vi "GetXYLocal.vi"(6 "Dummy Ref":refnum<vi>, 8 "error in (no error)":errorcluster, 10 "Global Mouse Coords":T1, 11 "Render Window in":refnum<class "Render Window.lvclass">) -> (0 "error out":errorcluster, 2 "Local Mouse Coords":T1, 3 "Render Window out":refnum<class "Render Window.lvclass">)   [LabVIEW 2015, in "Render Window.lvclass"]
uses:
  Render Window.lvclass
  3D Scene/Mouse Coords.ctl
  Render Window.lvclass/Render Window.ctl
  Input/Input.lvclass
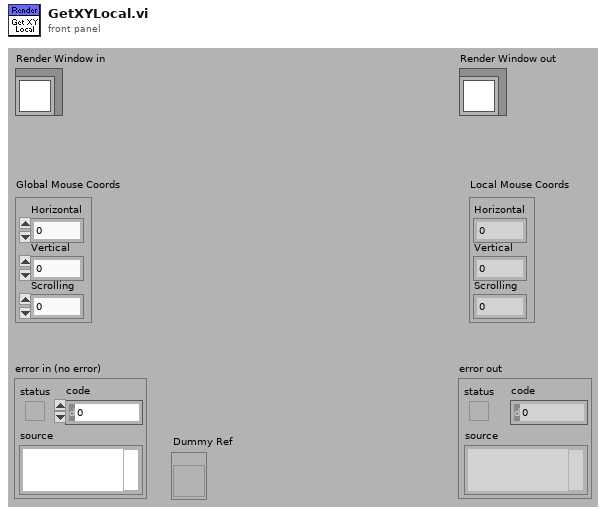
[diagram p1: front panel]
types:
  T1 = typedef "Input.lvclass/Mouse Coords.ctl" = cluster{"Horizontal":i32, "Vertical":i32, "Scrolling":i32}
  T2 = typedef "LVRectTypeDef.ctl" = cluster{"Left":i16, "Top":i16, "Right":i16, "Bottom":i16}
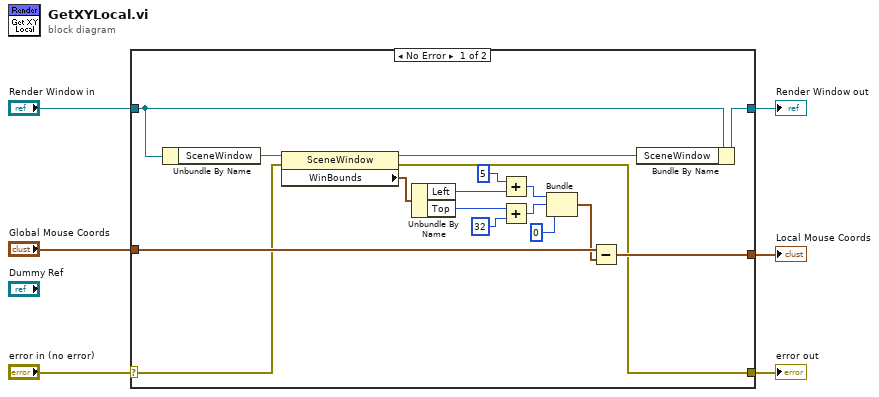
[diagram p0: block diagram]
diagram:
  n1 = case shown="No Error" "error in (no error)" {
    selector: "error in (no error)" -> [w10 w26]
    tunnel: [w9 w26] -> w5
    tunnel: [w22 w25] -> w3
    tunnel: "Render Window in" -> [w23 w25]
    tunnel: "Global Mouse Coords" -> [w13 w24]
    tunnel: [w12 w24] -> w1
    frame No Error {
      n2 = Unbundle By Name(w23) -> ("SceneWindow"=w21:refnum<vi>)
      n3 = property class="SceneWindow"(reference=w21, error in=w10) -> (reference out=w11:refnum<vi>, error out=w9:errorcluster, "WinBounds"=w20:T2)
      n4 = Unbundle By Name(w20) -> ("Left"=w19:i16, "Top"=w17:i16)
      n5 = Add(x=i16 5, y=w19) -> (x+y=w15:i16)
      n6 = Add(x=w17, y=i16 32) -> (x+y=w14:i16)
      n7 = Bundle(w15, w14, "y"=i16 0) -> (w7:cluster{i16, i16, "y":i16})  [unwired: 1 out]
      n8 = Subtract(x=w13, y=w7) -> (x-y=w12:T1)
      n9 = Bundle By Name(cluster=w23, "SceneWindow"=w11) -> (w22:refnum<class "Render Window.lvclass">)
    }
    frame Error {
    }
  }
  "error out" <- w5
  "Render Window out" <- w3
  "Local Mouse Coords" <- w1
